vi "Read Power Meter.lvclass.vi"(11 "Power Meter GUI in":refnum<class "Power Meter GUI.lvclass">) -> (2 "Power Meters":refnum<class "Power Meter.lvclass">[](array[class]), 3 "Power Meter GUI out":refnum<class "Power Meter GUI.lvclass">)   [LabVIEW 2020, in "Power Meter GUI.lvclass"]
uses:
  Power Meter GUI.lvclass
  Instruments/Power Meter/Power Meter.lvclass
  Power Meter GUI.lvclass/Power Meter GUI.ctl
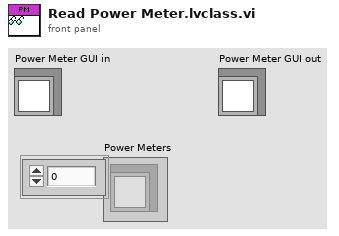
[diagram p1: front panel]
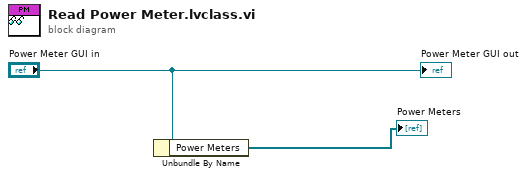
[diagram p0: block diagram]
diagram:
  n1 = Unbundle By Name("Power Meter GUI in") -> ("Power Meters"=→"Power Meters":refnum<class "Power Meter.lvclass">[])
  "Power Meter GUI out" <- "Power Meter GUI in"
